vi "Configure Output Off Behavior.vi"(8 "error in (no error)":errorcluster, 10 "Output Off Behavior (0: Normal)":u16(ring) items=["Normal", "High Impedance", "Zero", "Guard"], 11 "VISA resource name":refnum<visa-resource-name>) -> (0 "error out":errorcluster, 3 "VISA resource name out":refnum<visa-resource-name>)   [LabVIEW 2017, in "Keithley 24XX.lvlib"]
doc: "Configures the instrument's behavior when the output is disabled."
uses:
  Keithley 24XX.lvlib
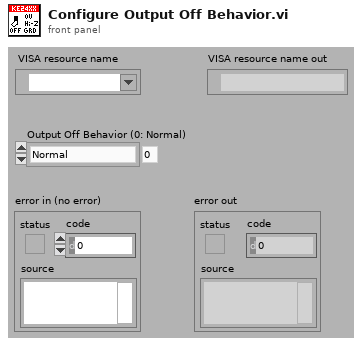
[diagram p1: front panel]
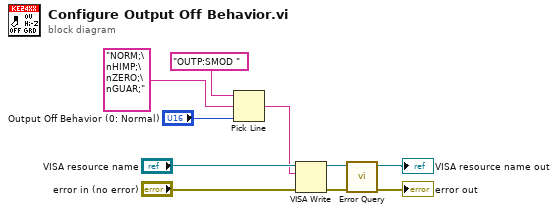
[diagram p0: block diagram]
diagram:
  n1 = Pick Line(string ("")="OUTP:SMOD ", multi-line string="NORM;\nHIMP;\nZERO;\nGUAR;", line index="Output Off Behavior (0: Normal)") -> (output string=w5:string)
  n2 = VISA Write(VISA resource name="VISA resource name", write buffer=w5, error in (no error)="error in (no error)") -> (VISA resource name out=w4:refnum<visa-resource-name>, error out=w1:errorcluster)  [unwired: 1 out]
  n3 = call "Error Query.vi"("error in (no error)"=w1, "VISA resource name"=w4) -> ("error out"=→"error out":errorcluster, "VISA resource name out"=→"VISA resource name out":refnum<visa-resource-name>)  [unwired: 6 in, 2 out]
